vi "6009 Simple LV71.vi"() -> ()   [LabVIEW 2020]
uses:
  <vilib>/DAQmx/read.llb/DAQmx Read.vi
  <vilib>/DAQmx/read.llb/DAQmx Read (Analog 1D Wfm NChan NSamp).vi
panel:
  in  "Channel B":tag
  in  "Channel A":tag
  out "path":path
  out "OriginWks":refnum<k7>
  out "Samples in Buffer (Scan Backlog)":u32
  out "Reading Fast Enough?":bool
  in  "Read Wait (ms)":dbl=200.0
  in  "Buffer Size":dbl=1000.0
  out "Waveforms":waveform(dbl)[](graph)
  in  "stop":bool
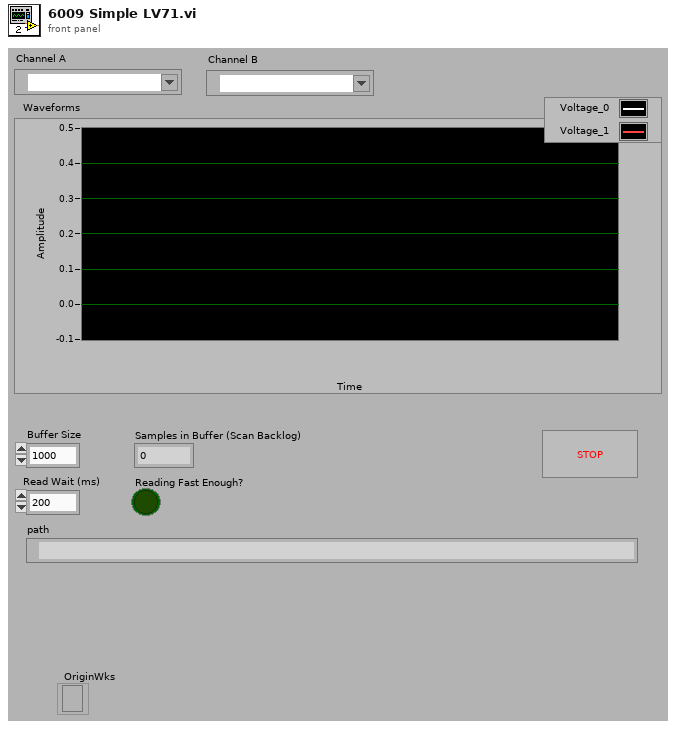
[diagram p1: front panel]
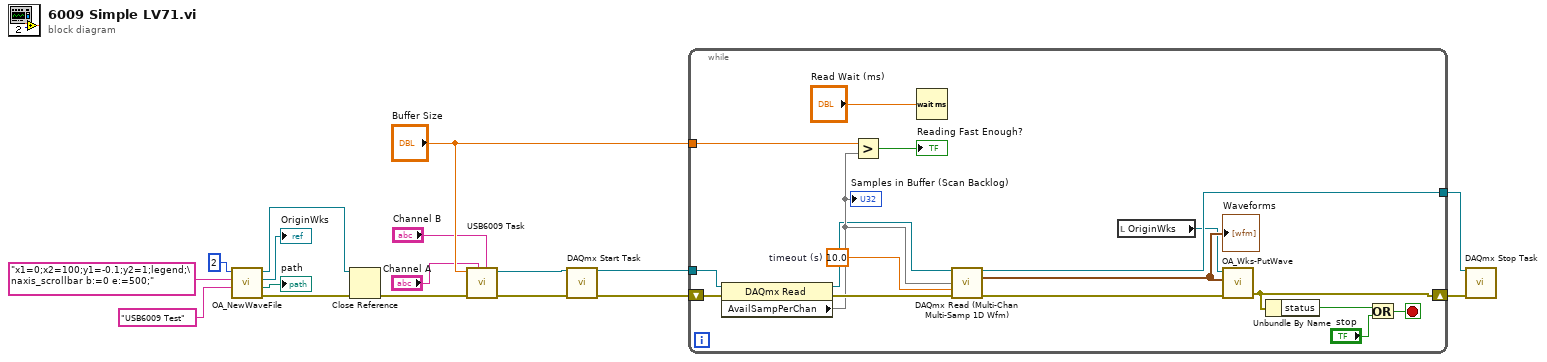
[diagram p0: block diagram]
diagram:
  n1 = call "OA_NewWaveFile.vi"("Origin file name"="USB6009 Test", "graph script"="x1=0;x2=100;y1=-0.1;y2=1;legend;\naxis_scrollbar b:=0 e:=500;", "number of columns"=2) -> ("error out"=w2:errorcluster, "path out"=→"path":path, "Origin.Worksheet"=→"OriginWks":refnum<k7>, "Origin.IOApplication"=w1:refnum<k7>)  [unwired: 5 in]
  n2 = Close Reference(reference=w1, error in (no error)=w2) -> (error out=w3:errorcluster)
  n3 = call "USB6009 Task.vi"("physical channels 2"="Channel B", "physical channels"="Channel A", "error in"=w3, "number of samples"="Buffer Size") -> ("error out"=w14:errorcluster, "task out"=w15:refnum<k21>)  [unwired: 6 in]
  n4 = call <vilib>:"DAQmx Start Task.vi"("task/channels in"=w15, "error in"=w14) -> ("task out"=w17:refnum<k21>, "error out"=w16:errorcluster)  [unwired: 12 in]
  n5 = while {
    tunnel: w17 -> [w29]
    tunnel: [w34] -> w7
    shift-right: [w18] -> w6
    shift-left: w16 -> [w28]
    tunnel: "Buffer Size" -> [w20]
    stop <- w32 stop-if-true
    w30 = 10.0  # timeout (s)
    n6 = property class="DAQmx Read"(reference=w29, error in=w28) -> (reference out=w24:refnum<k21>, error out=w27:errorcluster, "AvailSampPerChan"=w26)
    "Samples in Buffer (Scan Backlog)" <- w26
    n7 = Greater?(x=w20, y=w26) -> (0:→"Reading Fast Enough?":bool)
    n8 = Wait (ms)(milliseconds to wait="Read Wait (ms)") -> ()  [unwired: 1 out]
    n9 = call-poly "DAQmx Read (Multi-Chan Multi-Samp 1D Wfm).vi"("task/channels in"=w24, "number of samples per channel"=w26, "timeout"=w30, "error in"=w27) -> ("task out"=w34:refnum<k21>, "data"=w23:waveform(dbl)[], "error out"=w22:errorcluster)  [unwired: 9 in]
    "Waveforms" <- w23
    n10 = local read "OriginWks"() -> (w21:refnum<k7>)
    n11 = call "OA_Wks-PutWave.vi"("Origin.Worksheet"=w21, "Dynamic Data"=w23, "error in (no error)"=w22) -> ("error IO"=w18:errorcluster)  [unwired: 3 in, 1 out]
    n12 = Unbundle By Name(w18) -> ("status"=w33:bool)
    n13 = Or(x=w33, y="stop") -> (x .or. y?=w32:bool)
  }
  n14 = call <vilib>:"DAQmx Stop Task.vi"("task/channels in"=w7, "error in"=w6) -> ()  [unwired: 12 in, 2 out]
